vi "rm.server.unreserve resource.vi"(8 "error in (no error)":errorcluster, 10 "Name in bitfile":string, 11 "Item Ref in":T1 format="%.0x") -> (0 "error out":errorcluster, 1 "found?":bool, 3 "Item Ref out":T1 format="%.0x")   [LabVIEW 2016, in "RM.Server.lvlib"]
uses:
  RM.Server.lvlib
  <vilib>/NI Veristand/Custom Device API/Custom Device Item Ref.ctl
  <vilib>/NI VeriStand/Custom Device API/Custom Device API.lvlib
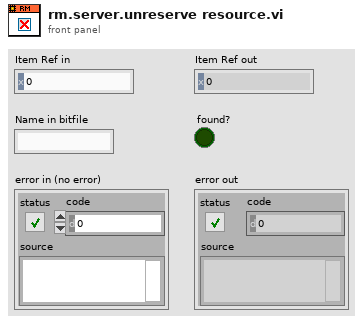
[diagram p1: front panel]
types:
  T1 = typedef "Custom Device API.lvlib/Custom Device Item Ref.ctl" = u64
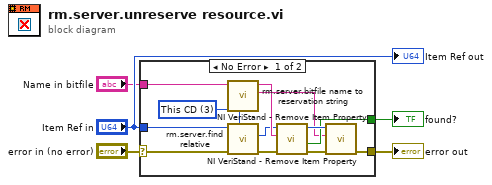
[diagram p0: block diagram]
diagram:
  n1 = case shown="No Error" "error in (no error)" {
    selector: "error in (no error)" -> [w14 w18]
    tunnel: [w11 w18] -> w4
    tunnel: "Item Ref in" -> [w15 _]
    tunnel: "Name in bitfile" -> [w12 _]
    tunnel: [w9 _] -> w1
    frame No Error {
      w16 = u16 3 items=["Targets", "Controller", "Custom Devices", "This CD", "This CD/Group", "This CD/Group/SubGroup"] ("Relative Type")
      n2 = call "rm.server.bitfile name to reservation string.vi"("Name in bitfile"=w12) -> ("Notes String"=w8:string, "Reservation String"=w7:string)  [unwired: 9 in]
      n3 = call "rm.server.find relative.vi"("Relative Type"=w16, "error in (no error)"=w14, "Item Ref in"=w15) -> ("error out"=w13:errorcluster, "Relative Item Ref Out"=w6:T1)  [unwired: 4 in, 3 out]
      n4 = call <vilib>:"NI VeriStand - Remove Item Property.vi"("error in (no error)"=w13, "Property Name"=w7, "Item Ref in"=w6) -> ("error out"=w17:errorcluster, "Removed"=w9:bool, "Item Ref out"=w10:T1)  [unwired: 6 in]
      n5 = call <vilib>:"NI VeriStand - Remove Item Property.vi"("error in (no error)"=w17, "Property Name"=w8, "Item Ref in"=w10) -> ("error out"=w11:errorcluster)  [unwired: 6 in, 2 out]
    }
    frame Error {
    }
  }
  "error out" <- w4
  "found?" <- w1
  "Item Ref out" <- "Item Ref in"
